vi "wind-dir-calc.vi"(11 "Analog Direction":dbl step=100.0) -> (2 "Ndir":T1=enum."NE", 3 "Wind Dir View":T2)   [LabVIEW 2024]
uses:
  controls/wind-dir-view.ctl
  controls/wind-directions.ctl
panel:
  out "Dir":T1=enum."NE"
  out "NW":bool
  out "SE":bool
  out "W":bool
  out "SW":bool
  out "S":bool
  out "E":bool
  out "NE":bool
  out "N":bool
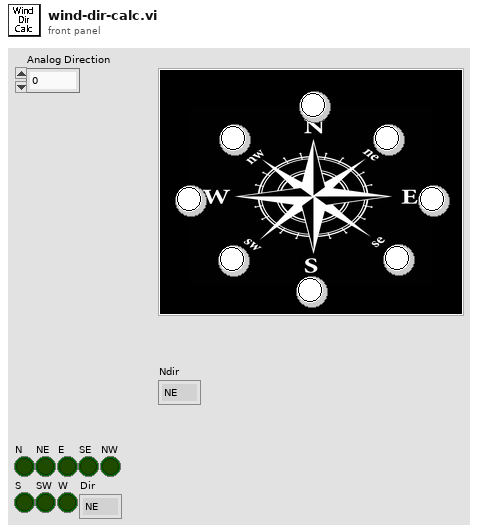
[diagram p1: front panel]
types:
  T1 = typedef "wind-directions.ctl" = enum16{"N", "NE", "E", "SE", "S", "SW", "W", "NW"}
  T2 = typedef "wind-dir-view.ctl" = cluster{"SE":bool, "SW":bool, "NE":bool, "NW":bool, "W":bool, "E":bool, "S":bool, "N":bool}
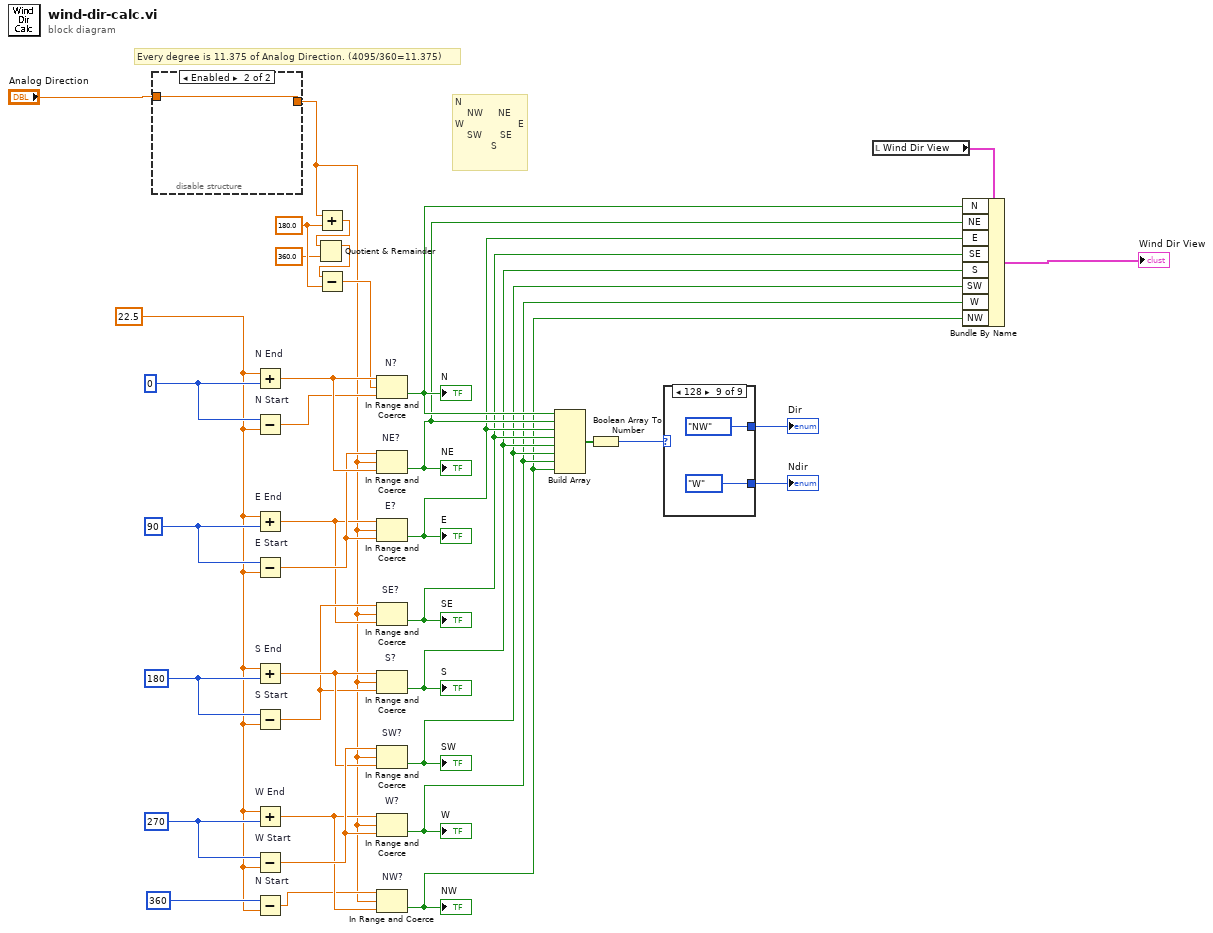
[diagram p0: block diagram]
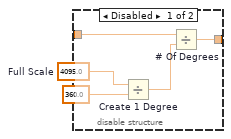
[diagram p2: hidden frame]
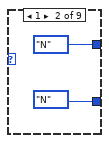
[diagram p4: hidden frame]
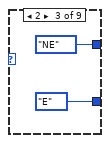
[diagram p5: hidden frame]
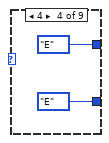
[diagram p6: hidden frame]
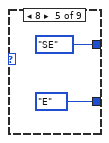
[diagram p7: hidden frame]
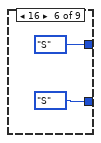
[diagram p8: hidden frame]
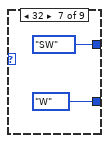
[diagram p9: hidden frame]
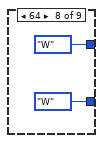
[diagram p10: hidden frame]
diagram:
  w16 = 22.5 ("Dir Offset")
  w3 = 180.0 ("y")
  w27 = 270 ("y")
  w26 = 180 ("y")
  w32 = 90 ("y")
  w33 = 0 ("y")
  # "Every degree is 11.375 of Analog Direction. (4095/360=11.375)"
  # "N\n    NW     NE\nW                  E\n    SW      SE\n            S"
  n1 = disable-structure shown="Enabled" {
    disable-tunnel: "Analog Direction" -> [w41 w42]
    disable-tunnel: [w40 w42] -> w14
    frame Disabled {
      w38 = 4095.0  # Full Scale
      n2 = Divide "Create 1 Degree"(x=w38, y=360.0) -> (x/y=w37:dbl)
      n3 = Divide "# Of Degrees"(x=w41, y=w37) -> (x/y=w40:dbl)
    }
    frame Enabled {
    }
  }
  n4 = Add "N End"(x=w16, y=w33) -> (x+y=w31:dbl)
  n5 = Subtract "N Start"(x=w33, y=w16) -> (x-y=w18:dbl)
  n6 = Add "E End"(x=w16, y=w32) -> (x+y=w24:dbl)
  n7 = Subtract "E Start"(x=w32, y=w16) -> (x-y=w30:dbl)
  n8 = Add "S End"(x=w16, y=w26) -> (x+y=w28:dbl)
  n9 = Subtract "S Start"(x=w26, y=w16) -> (x-y=w25:dbl)
  n10 = Add "W End"(x=w16, y=w27) -> (x+y=w23:dbl)
  n11 = Subtract "W Start"(x=w27, y=w16) -> (x-y=w29:dbl)
  n12 = Subtract "N Start"(x=360 ("y"), y=w16) -> (x-y=w15:dbl)
  n13 = Add(x=w14, y=w3) -> (x+y=w5:dbl)
  n14 = Quotient & Remainder(x=w5, y=360.0) -> (x-y*floor(x/y)=w4:dbl)  [unwired: 1 out]
  n15 = Subtract(x=w4, y=w3) -> (x-y=w19:dbl)
  n16 = In Range and Coerce "N?"(upper limit=w31, x=w19, lower limit=w18) -> (In Range?=w13:bool)  [unwired: 1 out]
  "N" <- w13
  n17 = In Range and Coerce "NE?"(upper limit=w30, x=w14, lower limit=w31) -> (In Range?=w12:bool)  [unwired: 1 out]
  "NE" <- w12
  n18 = In Range and Coerce "E?"(upper limit=w24, x=w14, lower limit=w30) -> (In Range?=w11:bool)  [unwired: 1 out]
  "E" <- w11
  n19 = In Range and Coerce "SE?"(upper limit=w25, x=w14, lower limit=w24) -> (In Range?=w10:bool)  [unwired: 1 out]
  "SE" <- w10
  n20 = In Range and Coerce "S?"(upper limit=w28, x=w14, lower limit=w25) -> (In Range?=w9:bool)  [unwired: 1 out]
  "S" <- w9
  n21 = In Range and Coerce "SW?"(upper limit=w29, x=w14, lower limit=w28) -> (In Range?=w8:bool)  [unwired: 1 out]
  "SW" <- w8
  n22 = In Range and Coerce "W?"(upper limit=w23, x=w14, lower limit=w29) -> (In Range?=w7:bool)  [unwired: 1 out]
  "W" <- w7
  n23 = In Range and Coerce "NW?"(upper limit=w15, x=w14, lower limit=w23) -> (In Range?=w6:bool)  [unwired: 1 out]
  "NW" <- w6
  n24 = Build Array(w13, w12, w11, w10, w9, w8, w7, w6) -> (w22:bool[])
  n25 = Boolean Array To Number(Boolean array=w22) -> (number=w21:u32)
  n26 = case shown="128" w21 {
    tunnel: [_ wind-directions."N" wind-directions."NE" wind-directions."E" wind-directions."SE" wind-directions."S" wind-directions."SW" wind-directions."W" wind-directions."NW"] -> w1
    tunnel: [_ wind-directions."N" wind-directions."E" wind-directions."E" wind-directions."E" wind-directions."S" wind-directions."W" wind-directions."W" wind-directions."W"] -> w20
    frame 0, Default {
    }
    frame 1 {
    }
    frame 2 {
    }
    frame 4 {
    }
    frame 8 {
    }
    frame 16 {
    }
    frame 32 {
    }
    frame 64 {
    }
    frame 128 {
    }
  }
  "Dir" <- w1
  "Ndir" <- w20
  n27 = local read "Wind Dir View"() -> (w36:T2)
  n28 = Bundle By Name(cluster=w36, "N"=w13, "NE"=w12, "E"=w11, "SE"=w10, "S"=w9, "SW"=w8, "W"=w7, "NW"=w6) -> (→"Wind Dir View":T2)
